vi "Keithley 2002 Calc1 Config.vi"(1 "a0 Coefficient":dbl step=1.0 format="%.6e", 2 "a1 Coefficient":dbl=1.0 step=1.0 format="%.6e", 3 "a2 Coefficient":dbl step=1.0 format="%.6e", 4 "error in":T1, 5 "percent target value":dbl=1.0 step=1.0 format="%.6e", 6 "calculation1 (none:2)":u16(ring)=2 items=["polynomial", "percent", "none"], 7 "GPIB address":string="16") -> (0 "error out":T1)   [LabVIEW 2020]
doc: "This VI is used to configure the setup for math calculation 1 which is either the Polynomial a2*x^2+a1*x+a0 or the percent calculation.\n\nTo read the results of the calculation, use the Calc Read VI."
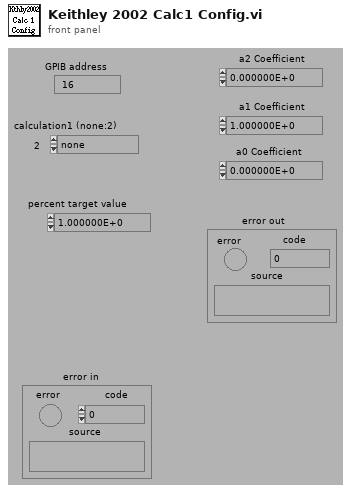
[diagram p1: front panel]
types:
  T1 = cluster{"error":bool, "code":i32, "source":string}
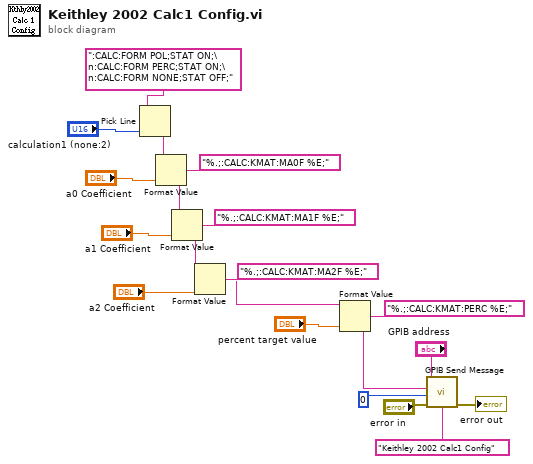
[diagram p0: block diagram]
diagram:
  n1 = Pick Line(multi-line string=":CALC:FORM POL;STAT ON;\n:CALC:FORM PERC;STAT ON;\n:CALC:FORM NONE;STAT OFF;", line index="calculation1 (none:2)") -> (output string=w12:string)  [unwired: 1 in]
  n2 = Format Value(string ("")=w12, format string="%.;:CALC:KMAT:MA0F %E;", value (0)="a0 Coefficient") -> (output string=w8:string)
  n3 = Format Value(string ("")=w8, format string="%.;:CALC:KMAT:MA1F %E;", value (0)="a1 Coefficient") -> (output string=w3:string)
  n4 = Format Value(string ("")=w3, format string="%.;:CALC:KMAT:MA2F %E;", value (0)="a2 Coefficient") -> (output string=w1:string)
  n5 = Format Value(string ("")=w1, format string="%.;:CALC:KMAT:PERC %E;", value (0)="percent target value") -> (output string=w5:string)
  n6 = call "GPIB Send Message.vi"("address string"="GPIB address", "write buffer"=w5, "source"="Keithley 2002 Calc1 Config", "write mode (set END:0)"=0, "error in"="error in") -> ("error out"=→"error out":T1)  [unwired: 2 in, 2 out]
